vi "SetRightPaneSize.vi"(8 "error in (no error)":errorcluster, 9 "Right Pane Size":i32, 10 "Front Panel":refnum<vi>, 11 "Splitters":T1) -> (0 "error out":errorcluster)   [LabVIEW 2022 SP3, in "PentaPanesLibrary.lvlib" / "PentaPanes.lvclass"]
uses:
  PentaPanes.lvclass
  SplittersCluster.ctl
panel:
  out "Bounds:Area Width 2":i32
  out "In Range?":bool
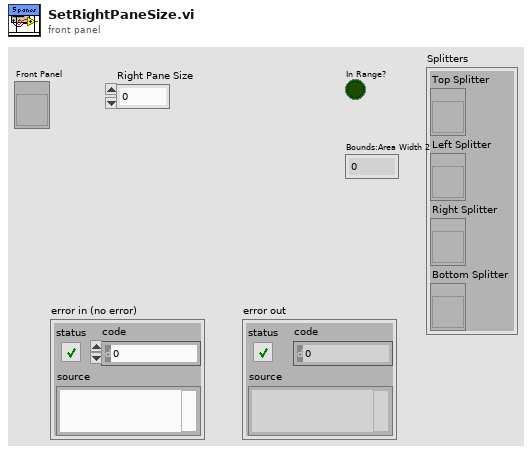
[diagram p1: front panel]
types:
  T1 = typedef "PentaPanesLibrary.lvlib/PentaPanes.lvclass/SplittersCluster.ctl" = cluster{"Top Splitter":refnum<vi>, "Left Splitter":refnum<vi>, "Right Splitter":refnum<vi>, "Bottom Splitter":refnum<vi>}
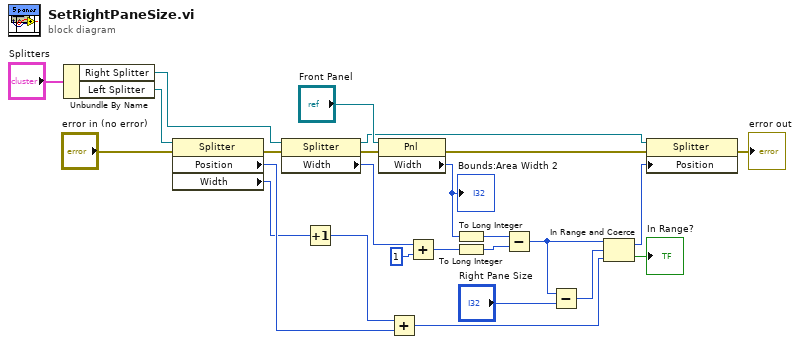
[diagram p0: block diagram]
diagram:
  n1 = Unbundle By Name("Splitters") -> ("Right Splitter"=w22:refnum<vi>, "Left Splitter"=w21:refnum<vi>)
  n2 = property class="Splitter"(reference=w21, error in="error in (no error)") -> (error out=w2:errorcluster, "Position"=w17:i32, "Width"=w6:u32)  [unwired: 1 out]
  n3 = property class="Splitter"(reference=w22, error in=w2) -> (reference out=w4:refnum<vi>, error out=w14:errorcluster, "Width"=w12:u32)
  n4 = Increment(x=w6) -> (x+1=w5:u32)
  n5 = property class="Pnl"(reference="Front Panel", error in=w14) -> (error out=w13:errorcluster, "Width"=w8:u32)  [unwired: 1 out]
  "Bounds:Area Width 2" <- w8
  n6 = Add(x=w5, y=w17) -> (x+y=w16:u32)
  n7 = Add(x=w12, y=1) -> (x+y=w10:u32)
  n8 = To Long Integer(number=w8) -> (32bit integer=w7:i32)
  n9 = To Long Integer(number=w10) -> (32bit integer=w9:i32)
  n10 = Subtract(x=w7, y=w9) -> (x-y=w15:i32)
  n11 = Subtract(x=w15, y="Right Pane Size") -> (x-y=w20:i32)
  n12 = In Range and Coerce(upper limit=w15, x=w20, lower limit=w16) -> (coerced(x)=w19:u32, In Range?=→"In Range?":bool)
  n13 = property class="Splitter"(reference=w4, error in=w13, "Position"=w19) -> (error out=→"error out":errorcluster)  [unwired: 1 out]
